vi "AMI1700eth_set_meas_mode.vi"(5 "int_samp":i8=15, 7 "mode":enum16{"CONT", "HOLD"}(ring), 8 "error in":errorcluster, 11 "conn_id_in":refnum<k5>) -> (0 "error out":errorcluster, 3 "conn_id_out":refnum<k5>)   [LabVIEW 2019]
panel:
  out "string_2":string
  out "string_1":string
  # "= Sampling interval in minute."
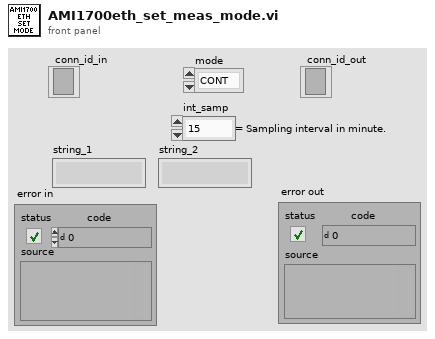
[diagram p1: front panel]
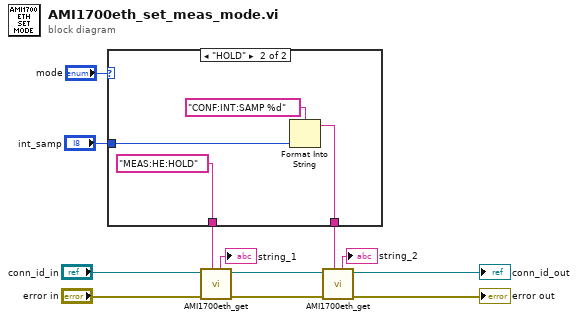
[diagram p0: block diagram]
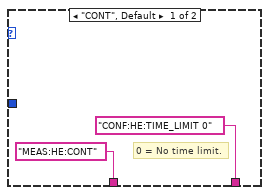
[diagram p2: hidden frame]
diagram:
  n1 = case shown="\"HOLD\"" "mode" {
    tunnel: ["MEAS:HE:CONT" "MEAS:HE:HOLD"] -> w4
    tunnel: ["CONF:HE:TIME_LIMIT 0" ("string in") w15] -> w3
    tunnel: "int_samp" -> [_ w17]
    frame "CONT", Default {
      # "0 = No time limit."
    }
    frame "HOLD" {
      n2 = Format Into String(format string="CONF:INT:SAMP %d" ("string in"), w17) -> (resulting string=w15:string)  [unwired: 2 in, 1 out]
    }
  }
  n3 = call "AMI1700eth_get.vi"("command"=w4, "error in"="error in", "conn_id_in"="conn_id_in") -> ("error out"=w8:errorcluster, "conn_id_out"=w9:refnum<k5>, "string"=→"string_1":string)  [unwired: 5 in, 1 out]
  n4 = call "AMI1700eth_get.vi"("command"=w3, "error in"=w8, "conn_id_in"=w9) -> ("error out"=→"error out":errorcluster, "conn_id_out"=→"conn_id_out":refnum<k5>, "string"=→"string_2":string)  [unwired: 5 in, 1 out]
